vi "Topo & GridSpectr_DriftCorrection_zSpec_v18.vi"(6 "Internal use":string, 7 "Grid param":T1 {"height (m)" format="%#_6p"; "width (m)" format="%#_6p"; "center Y (m)" format="%#_6p"; "center X (m)" format="%#_6p"}, 8 "Error in (no error)":errorcluster, 9 "Points Y/Index Y":i32, 10 "Points X/Index X":i32, 11 "Method":enum16{"init", "run", "end"}(ring)=enum."end") -> (0 "Error out":errorcluster)   [LabVIEW 2014]
doc: "Example of a measurement VI to be used in the \"Experiments on a Grid\" tool as external VI.\n\nThis example measure the topography and spectroscopy data. The spectroscopy measurements are taken on a subgrid. The data are saved to a sxm and a binary file.\n\n- Nanonis Programming Interface -"
uses:
  <userlib>/Nanonis Prog Interface V5/Scan/Grid/GridPatternGet.vi
  <userlib>/Nanonis Prog Interface V5/Scan/Grid/LinePatternGet.vi
  <userlib>/Nanonis Prog Interface V5/Nanonis Prog Interface.lvlib
panel:
  in  "MultiGrid":bool
  in  "PLL ON/OFF":bool
  in  "Spectroscopy":u16(ring) items=["Bias", "zSpec"]
  in  "autoStop":bool
  in  "trigger 2 >Hz":sgl format="%#_6p"
  in  "trigger1 < Hz":sgl format="%#_6p"
  out "zFile":refnum<file>
  out "last z adjustment":sgl format="%#_6p"
  in  "during Spec Bias (V)":sgl format="%#_5p"
  in  "type":u16(ring)=1 items=["Line", "Grid"]
  in  "readjust setpoint every":i32=4
  in  "Correct Drift":bool=TRUE
  in  "Email when finished":string="cornelius.krull@monash.edu"
  in  "STS z offset":dbl format="%#_6p"
  out "ETA":timestamp
  out "remaining":dbl format="%<%H:%M:%S>t"
  out "Progress":u8(slide) scale=0.0..100.0 scale format="%#.1g"
  out "total Points":i32
  in  "preSTS delay [ms]":u32=500
  in  "ref Bias":dbl=0.02 format="%#_6p"
  in  "Imaging Bias":dbl=0.02 format="%#_6p"
  in  "max applied Drift Correction":i32=20 min=1 max=100 step=1 format="%.0p"
  in  "Correlate":u16(ring) items=["first Frame", "successive Frames"]
  out "Topo Images taken":i32=14
  in  "Increment":i32=40
  in  "Threshold":i32=2 min=1 step=1
  in  "tip Speed (m/s)":sgl=2e-09 format="%.2p"
  out "X drift":i32
  out "Y drift":i32
  out "Last Drift detected":i32=40
  in  "MaxImagesBack":i32=40
  in  "Channel index (0-23)":u8(ring) items=["Current"=0, "Z (m)"=14]
  in  "File name":string="symmetric_node"
  in  "ref Current":dbl=5e-12 format="%#_6p"
  in  "Imaging Current":dbl=5e-12 format="%#_6p"
  in  "zdrift \nDuration (s)":dbl
  in  "Correct z drift":bool
  out "Status":string="finishing"
  in  "Drift correction Pixels":i32=256 caption="Topo Pixels"
  out "Y Offset":dbl format="%#_6p"
  out "X Offset":dbl format="%#_6p"
  out "Points taken":dbl=14.0
  in  "Drift Correction every":i32=40
  # "z Spectroscopy"
  # "GRID points"
  # "Increase this if no Drift was detected for \na certain number of images"
  # "%"
  # "time (HH:MM:SS)"
  # "images back"
  # "% of image size"
  # "RUN smart tilt before starting the GRID\nImg Angle = 0\nmove tip to reference point for tip height"
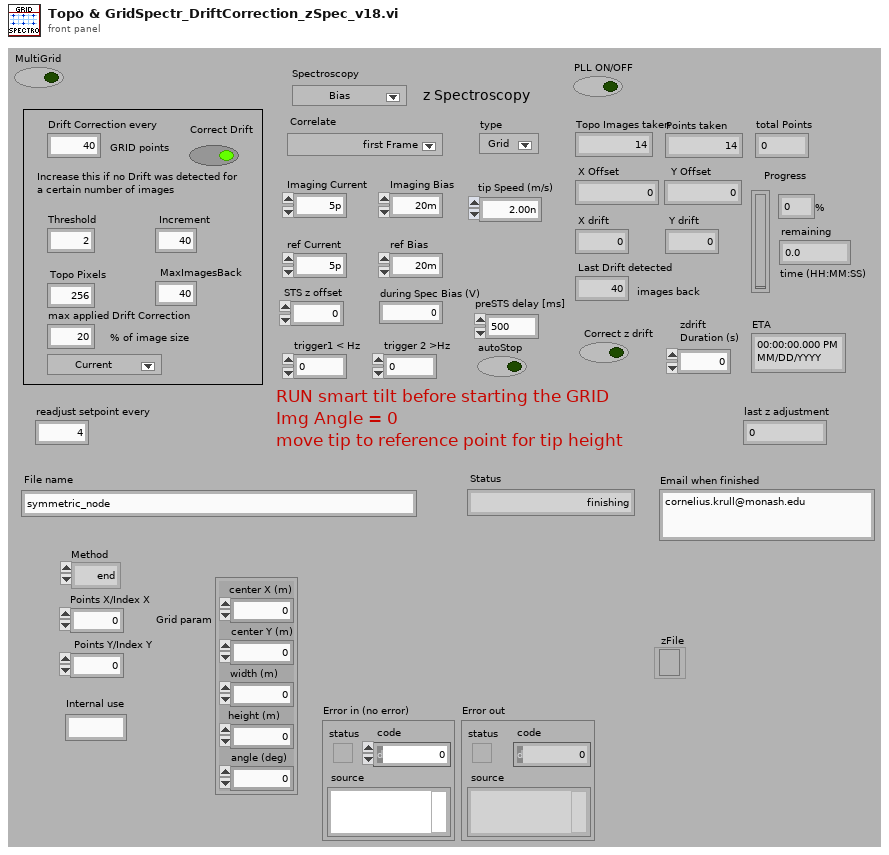
[diagram p1: front panel]
types:
  T1 = cluster{"center X (m)":sgl, "center Y (m)":sgl, "width (m)":sgl, "height (m)":sgl, "angle (deg)":sgl}
  T2 = enum16{"open", "replace", "create", "open or create", "replace or create", "replace or create with confirmation"}
  T3 = cluster{"Drift correction Pixels":i32, "Imaging Current":dbl, "STS Current":dbl, "MaxImagesBack":i32, "tip Speed (m/s)":sgl, "Threshold":i32, "Increment":i32, "Correlate":u16, "max applied Drift Correction":i32, "Imaging Bias":dbl, "Move Current":dbl, "Move Bias":dbl, "STS Bias":dbl, "preSTS delay [ms]":u32, "STS z offset":dbl, "Correct Drift":bool, "Lockin ON/OFF":bool}
  T4 = cluster{"x(m)":sgl, "y(m)":sgl, "Text":string, "Color":u32}
  T5 = cluster{"Z averaging time (s)":sgl, "Z offset (m)":sgl, "Initial settling time (s)":sgl}
  T6 = cluster{"center X":sgl, "center Y":sgl, "angle":sgl, "width":sgl, "height":sgl, "# pixels":i32, "# lines":i32}
  T7 = cluster{"Name":string, "Calibration":sgl, "Offset":sgl, "Channel index":i32}[]
  T8 = cluster{"up/down":bool, "time/line":sgl, "start time":timestamp, "end time":timestamp}
  T9 = cluster{"X (m)":sgl, "Y (m)":sgl, "Text":string, "Color":u32, "Visible":bool}[]
  T10 = cluster{"Max. slew rate (V/s)":sgl, "Settling time (s)":sgl, "Integration time (s)":sgl}
  T11 = cluster{"End settling time (s)":sgl, "Z control time (s)":sgl}
  T12 = cluster{"Z averaging time (s)":sgl, "Initial settling time (s)":sgl}
  T13 = cluster{"Max. slew rate (m/s)":sgl, "Settling time (s)":sgl, "Integration time (s)":sgl}
  T14 = cluster{"Points X/Index X":i32, "Points Y/Index Y":i32}
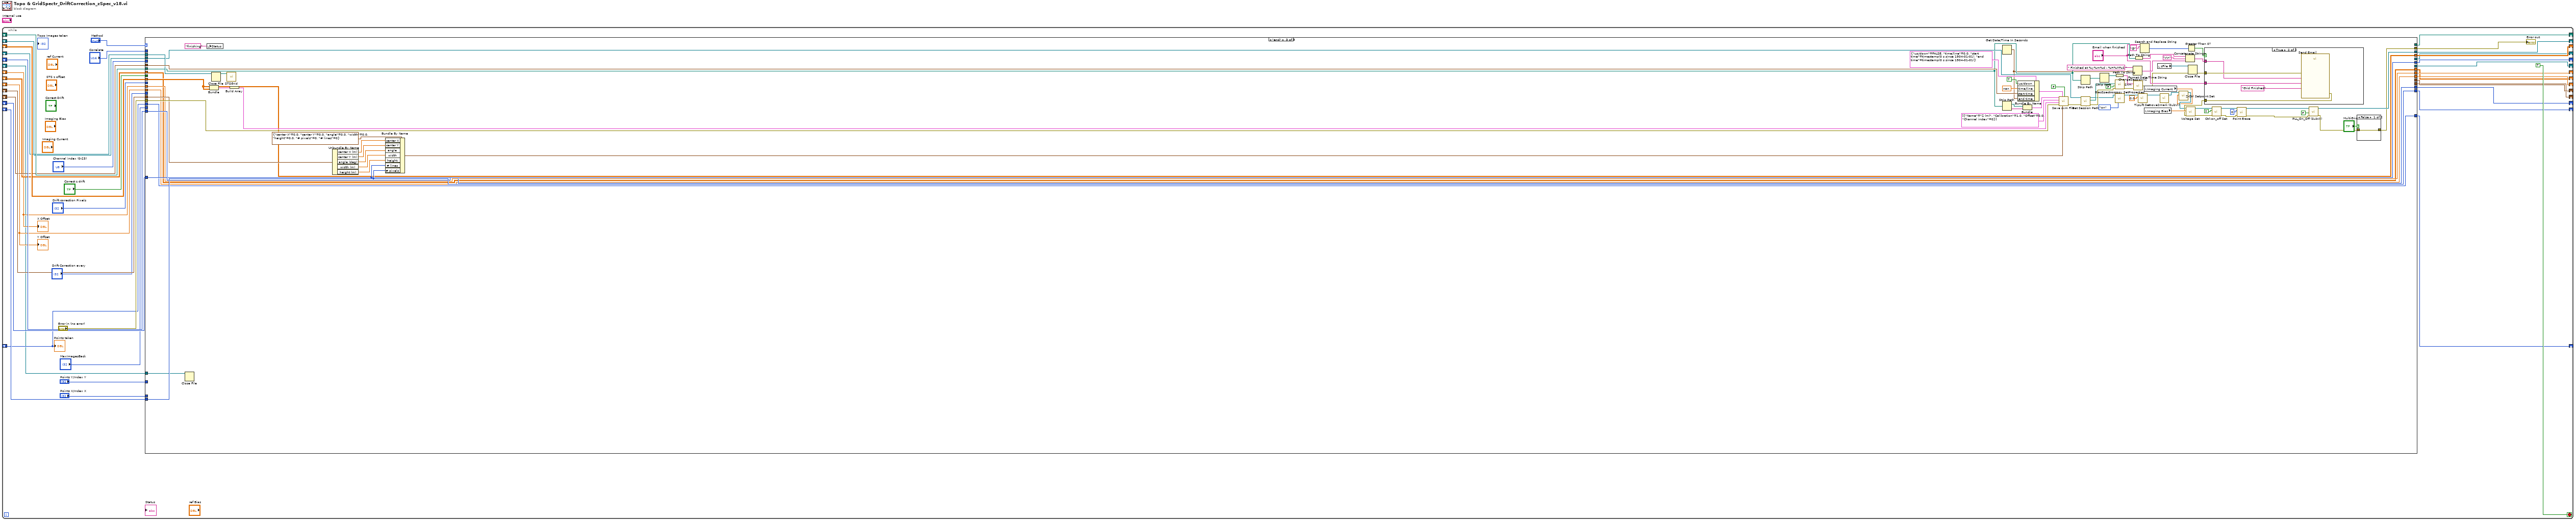
[diagram p0: block diagram]
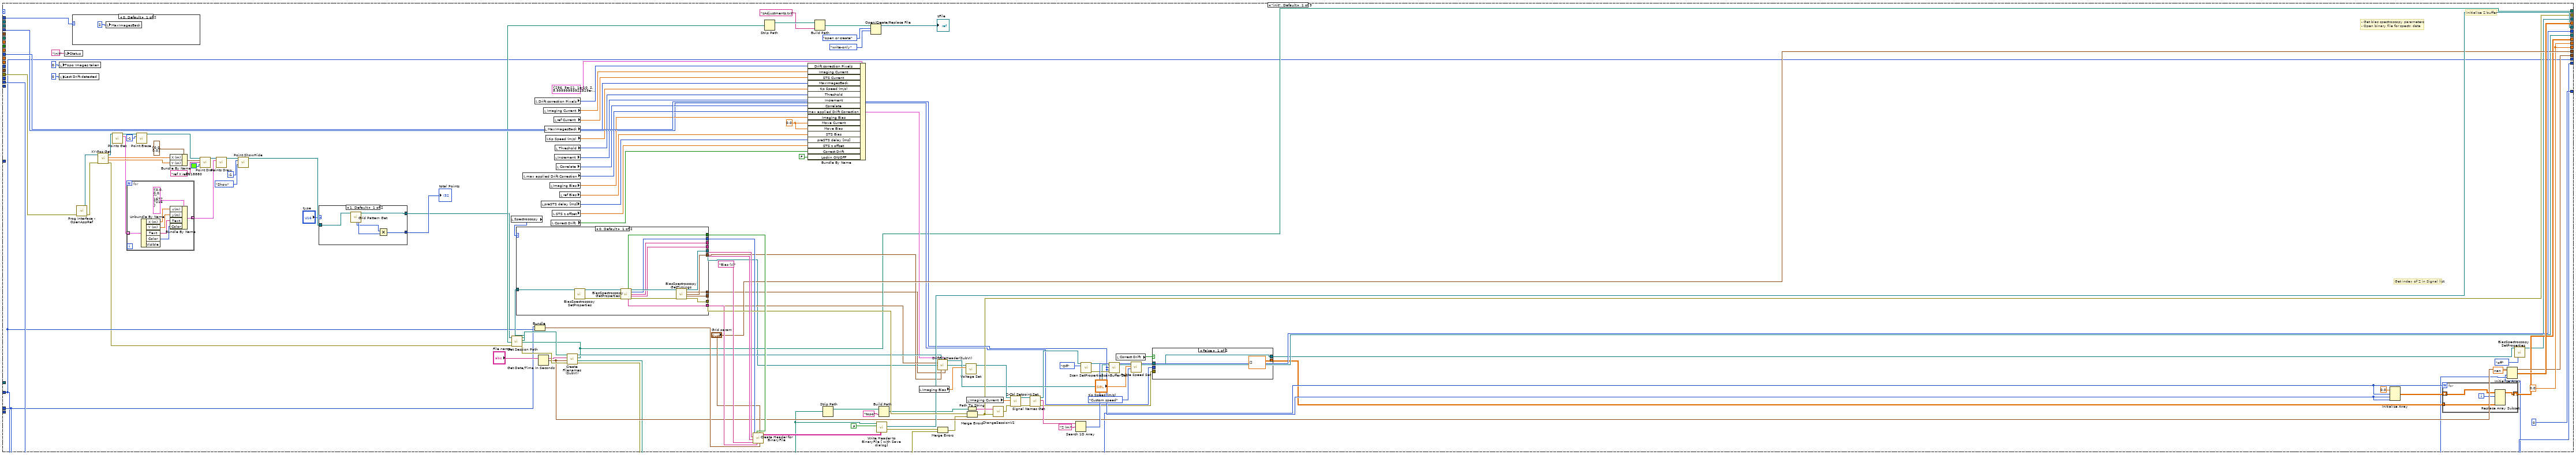
[diagram p2: hidden frame]
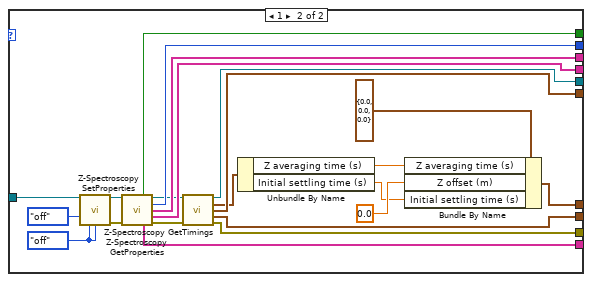
[diagram p3: hidden frame]
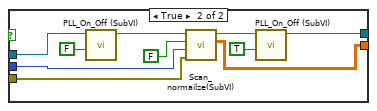
[diagram p4: hidden frame]
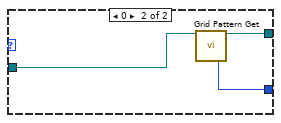
[diagram p5: hidden frame]
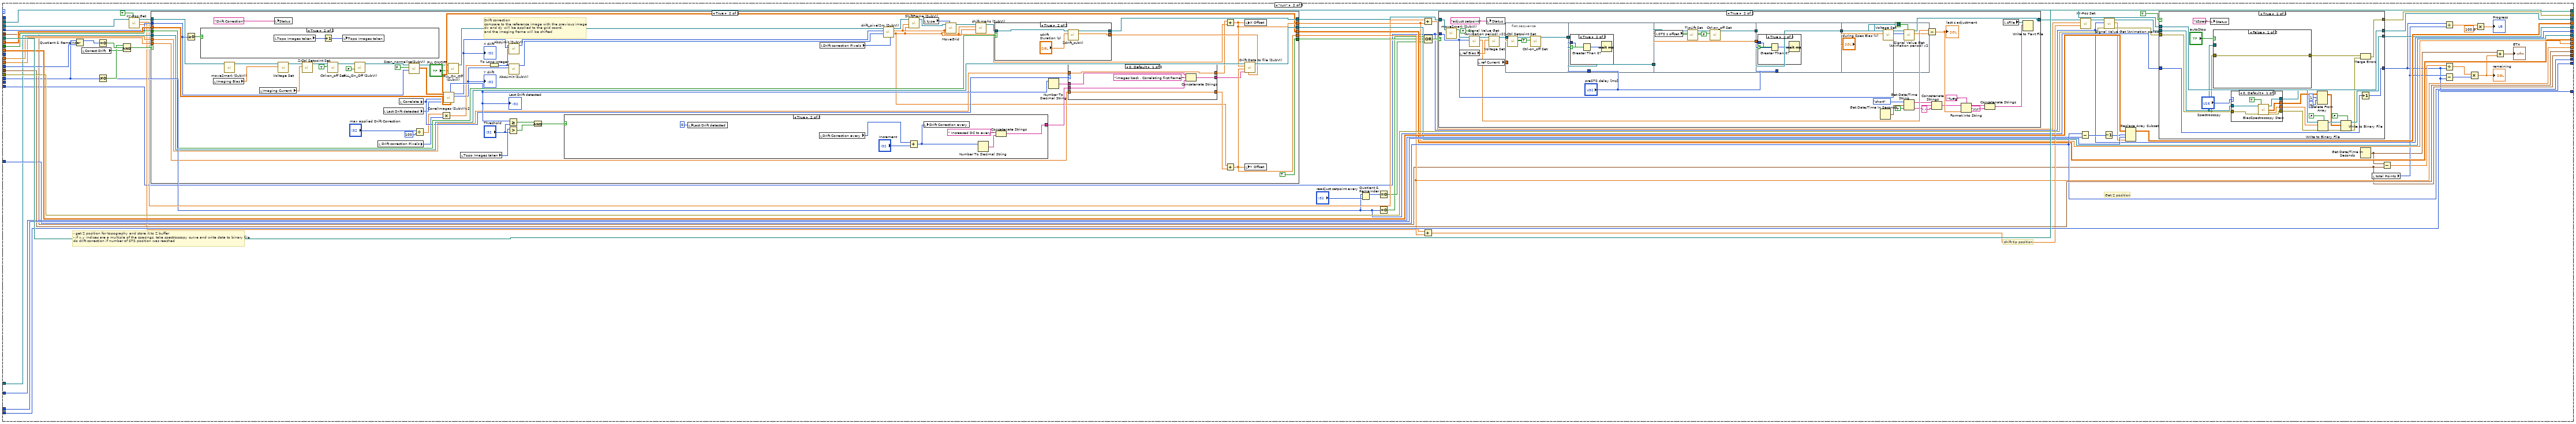
[diagram p7: hidden frame]
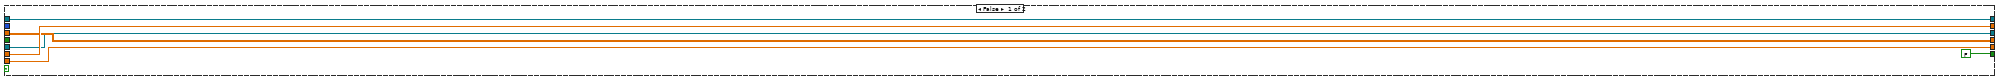
[diagram p11: hidden frame]
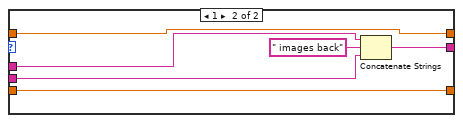
[diagram p12: hidden frame]
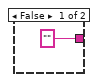
[diagram p14: hidden frame]
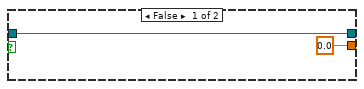
[diagram p15: hidden frame]
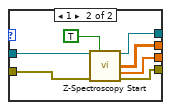
[diagram p17: hidden frame]
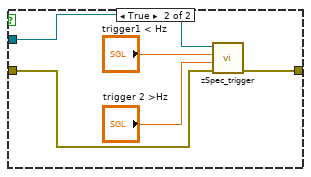
[diagram p18: hidden frame]
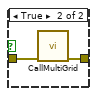
[diagram p19: hidden frame]
diagram:
  n1 = while {
    shift-right: [w21] -> _
    shift-left: _ -> [w38]
    shift-right: [w33] -> _
    shift-left: _ -> [w32]
    shift-right: [w30] -> _
    shift-left: _ -> [w31]
    shift-right: [w29] -> _
    shift-left: _ -> [w28]
    shift-right: [w27] -> _
    shift-left: _ -> [w26]
    shift-right: [w25] -> _
    shift-left: _ -> [w24]
    shift-right: [w23] -> _
    shift-left: _ -> [w22]
    shift-right: [w20] -> _
    shift-left: _ -> [w19]
    shift-right: [w18] -> _
    shift-left: _ -> [w17]
    shift-right: [w16] -> _
    shift-left: _ -> [w9]
    shift-right: [w15] -> _
    shift-left: _ -> [w8]
    shift-right: [w14] -> _
    shift-left: _ -> [w11]
    shift-right: [w13] -> _
    shift-left: _ -> [w10]
    shift-right: [w6] -> _
    shift-left: _ -> [w5]
    stop <- TRUE stop-if-true
    n2 = case shown="\"end\"" "Method" {
      tunnel: [w60 w296 _] -> w21
      tunnel: w38 -> [_ w296 w530]
      tunnel: "Error in (no error)" -> [w136 w289 w560]
      tunnel: [w116 w295 w498] -> w36
      tunnel: "Points X/Index X" -> [w53 w290 _]
      tunnel: "Points Y/Index Y" -> [w52 w283 _]
      tunnel: [w162 w293 w549] -> w33
      tunnel: w32 -> [_ w294 w549]
      tunnel: w31 -> [_ w292 w542]
      tunnel: [w154 w291 _] -> w30
      tunnel: [w152 w233 w572] -> w29
      tunnel: w28 -> [_ w233 w572]
      tunnel: [w105 w276 w507] -> w27
      tunnel: w26 -> [_ w260 w535]
      tunnel: ["Grid param" w286 _] -> w25
      tunnel: w24 -> [_ w286 w559]
      tunnel: [w134 w251 _] -> w23
      tunnel: w22 -> [_ w251 w567]
      tunnel: [w52 w284 w550] -> w20
      tunnel: w19 -> [_ w284 w550]
      tunnel: [w53 w285 w551] -> w18
      tunnel: w17 -> [_ w285 w551]
      tunnel: [w145 w266 w548] -> w16
      tunnel: [w145 w271 w546] -> w15
      tunnel: [w130 w265 w543] -> w14
      tunnel: [0 w249 w547] -> w13
      tunnel: w10 -> [_ w235 w547]
      tunnel: "Drift Correction every" -> [_ w279 _]
      tunnel: w11 -> [_ w270 w543]
      tunnel: w9 -> [_ w277 w548]
      tunnel: w8 -> [_ w263 w546]
      tunnel: "Drift correction Pixels" -> [w129 _ _]
      tunnel: [w102 w268 _] -> w6
      tunnel: w5 -> [_ w269 w544]
      tunnel: "Correct z drift" -> [_ w267 _]
      tunnel: "Channel index (0-23)" -> [w84 w264 _]
      tunnel: "MaxImagesBack" -> [w128 _ _]
      tunnel: "Correlate" -> [w112 _ _]
      frame "init", Default {
        w62 = 0.0 ("Move Current")
        w145 = 0.0
        # "- Get bias spectroscopy parameters\n- Open binary file for spectr. data"
        # "initialize Z buffer"
        # "Get index of Z in Signal list"
        n3 = local write "Topo Images taken"(0 ("Images taken")) -> ()
        n4 = local write "Last Drift detected"(0 ("Last Drift detected")) -> ()
        n5 = local write "Status"("init" ("Status")) -> ()
        n6 = case shown="0, Default" w112 {
          frame 0, Default {
            n7 = local write "MaxImagesBack"(2 ("StepsBack")) -> ()
          }
          frame 1 {
          }
        }
        n8 = call <userlib>:"Prog Interface - OpenAppRef.vi"("Error in (no error)"=w136) -> ("Error out"=w80:errorcluster, "Application reference"=w81:refnum<vi>)  [unwired: 5 in]
        n9 = call <userlib>:"XY-Pos Get.vi"("error in (no error)"=w80, "Application ref in"=w81) -> ("error out"=w49:errorcluster, "Y (m)"=w74:sgl, "X (m)"=w75:sgl, "Application ref out"=w45:refnum<vi>)  [unwired: 5 in]
        n10 = call <userlib>:"Points Get.vi"("Application ref in"=w45) -> ("Application ref out"=w44:refnum<vi>, "Points"=w46:T9)  [unwired: 12 in, 1 out]
        n11 = for {
          tunnel: w46 -> [w169] mode=indexing
          tunnel: [w163] -> w41 mode=indexing
          n12 = Unbundle By Name(w169) -> ("X (m)"=w167:sgl, "Y (m)"=w166:sgl, "Text"=w165:string, "Color"=w164:u32)  [unwired: 1 out]
          n13 = Bundle By Name(cluster=T4 {"x(m)"=0.0, "y(m)"=0.0, "Text"="", "Color"=16777216} ("Point"), "x(m)"=w167, "y(m)"=w166, "Text"=w165, "Color"=w164) -> (w163:T4)
        }
        n14 = call <userlib>:"Point Erase.vi"("Application ref in"=w44, "Point index (-1=All points)"=-1) -> ("Application ref out"=w67:refnum<vi>)  [unwired: 12 in, 1 out]
        n15 = Bundle By Name(cluster=cluster{"X (m)":sgl, "Y (m)":sgl} {"X (m)"=0.0, "Y (m)"=0.0} ("Point Coordinates"), "X (m)"=w75, "Y (m)"=w74) -> (w76:cluster{"X (m)":sgl, "Y (m)":sgl})
        n16 = call <userlib>:"Point Draw.vi"("Application ref in"=w67, "Point Coordinates"=w76, "Text"="ref X ref", "Color"=u32 6618880) -> ("Application ref out"=w43:refnum<vi>)  [unwired: 10 in, 1 out]
        n17 = call <userlib>:"Points Draw.vi"("Application ref in"=w43, "Points Configuration"=w41) -> ("Application ref out"=w42:refnum<vi>)  [unwired: 12 in, 1 out]
        n18 = call <userlib>:"Point ShowHide.vi"("Application ref in"=w42, "Point index (-1=All points)"=-1, "Show/Hide"=enum16{"Show", "Hide"}."Show") -> ("Application ref out"=w70:refnum<vi>)  [unwired: 11 in, 1 out]
        n19 = case shown="1, Default" "type" {
          tunnel: [w223 w226] -> w48
          tunnel: [w220 w224] -> w106
          tunnel: w70 -> [w219 w225]
          frame 1, Default {
            n20 = call-poly <userlib>:"Grid Pattern Get.vi"("Application ref in"=w219) -> ("Points Y"=w221:i32, "Points X"=w222:i32, "Application ref out"=w223:refnum<vi>)  [unwired: 10 in, 6 out]
            n21 = Multiply(x=w221, y=w222) -> (x*y=w220:i32)
          }
          frame 0 {
            n22 = call-poly <userlib>:"Grid Pattern Get.vi"("Application ref in"=w225) -> ("Points"=w224:i32, "Application ref out"=w226:refnum<vi>)  [unwired: 12 in, 5 out]
          }
        }
        "total Points" <- w106
        n23 = local read "Spectroscopy"() -> (w50:u16)
        n24 = call <userlib>:"Get Session Path.vi"("error in (no error)"=w49, "Application ref in"=w48) -> ("error out"=w135:errorcluster, "Session path"=w122:path, "Application ref out"=w114:refnum<vi>)  [unwired: 7 in]
        n25 = case shown="0, Default" w50 {
          tunnel: [w171 w206] -> w158
          tunnel: [w174 w205] -> w156
          tunnel: [w178 w192] -> w155
          tunnel: [w173 w204] -> w151
          tunnel: [w172 w203] -> w149
          tunnel: [w175 w202] -> w148
          tunnel: w114 -> [w180 w195]
          tunnel: [w177 w200] -> w73
          tunnel: [w176 w199] -> w72
          tunnel: [w170 w185] -> w47
          tunnel: [w179 w198] -> w51
          frame 0, Default {
            n26 = call <userlib>:"BiasSpectroscopy SetProperties.vi"("Application ref in"=w180) -> ("Application ref out"=w184:refnum<vi>, "Error out"=w183:errorcluster)  [unwired: 13 in]
            n27 = call <userlib>:"BiasSpectroscopy GetProperties.vi"("Application ref in"=w184, "Error in (no error)"=w183) -> ("Backward sweep"=w171:bool, "Application ref out"=w182:refnum<vi>, "Number of points"=w172:i32, "Channels"=w175:string[], "Parameters"=w174:string[], "Fixed parameters"=w173:string[], "Error out"=w181:errorcluster)  [unwired: 5 in, 2 out]
            n28 = call <userlib>:"BiasSpectroscopy GetTimings.vi"("Application ref in"=w182, "Error in (no error)"=w181) -> ("Application ref out"=w179:refnum<vi>, "Initialization"=w170:T5, "Sweep Timing"=w176:T10, "End of Sweep"=w177:T11, "Error out"=w178:errorcluster)  [unwired: 9 in]
          }
          frame 1 {
            w197 = enum16{"no change", "on", "off"}."off" ("Save dialog")
            n29 = call <userlib>:"Z-Spectroscopy SetProperties.vi"("Application ref in"=w195, "Autosave"=enum16{"no change", "on", "off"}."off" ("Autosave (no change)"), "Save dialog"=w197, "Save all sweeps (no change)"=w197) -> ("Application ref out"=w194:refnum<vi>, "error out"=w193:errorcluster)  [unwired: 10 in]
            n30 = call <userlib>:"Z-Spectroscopy GetProperties.vi"("Application ref in"=w194, "error in (no error)"=w193) -> ("Backward sweep"=w206:bool, "Application ref out"=w201:refnum<vi>, "Number of points"=w203:i32, "Channels"=w202:string[], "Parameters"=w205:string[], "Fixed parameters"=w204:string[], "error out"=w191:errorcluster)  [unwired: 6 in, 1 out]
            n31 = call <userlib>:"Z-Spectroscopy GetTimings.vi"("Application ref in"=w201, "Error in (no error)"=w191) -> ("Application ref out"=w198:refnum<vi>, "Initialization"=w186:T12, "Sweep Timing"=w199:T13, "End of Sweep"=w200:T11, "Error out"=w192:errorcluster)  [unwired: 9 in]
            n32 = Unbundle By Name(w186) -> ("Z averaging time (s)"=w188:sgl, "Initial settling time (s)"=w189:sgl)
            n33 = Bundle By Name(cluster=T5 {"Z averaging time (s)"=0.0, "Z offset (m)"=0.0, "Initial settling time (s)"=0.0} ("Initialization"), "Z averaging time (s)"=w188, "Z offset (m)"=sgl 0.0, "Initial settling time (s)"=w189) -> (w185:T5)
          }
        }
        n34 = local read "max applied Drift Correction"() -> (w90:i32)
        n35 = local read "Drift correction Pixels"() -> (w98:i32)
        n36 = Bundle("Points X/Index X"=w53, "Points Y/Index Y"=w52) -> (w157:T14)  [unwired: 1 in]
        n37 = Get Date/Time In Seconds() -> (seconds since 1Jan1904=w134:timestamp)
        n38 = local read "preSTS delay [ms]"() -> (w87:u32)
        n39 = local read "Imaging Current"() -> (w97:dbl)
        n40 = local read "MaxImagesBack"() -> (w94:i32)
        n41 = local read "tip Speed (m/s)"() -> (w95:sgl)
        n42 = local read "Imaging Bias"() -> (w89:dbl)
        n43 = local read "Correct Drift"() -> (w85:bool)
        n44 = local read "STS z offset"() -> (w86:dbl)
        n45 = local read "ref Current"() -> (w96:dbl)
        n46 = local read "Increment"() -> (w92:i32)
        n47 = local read "Threshold"() -> (w93:i32)
        n48 = local read "Correlate"() -> (w91:u16)
        n49 = local read "ref Bias"() -> (w88:dbl)
        n50 = call "Create Filenames (SubVI).vi"("error in (no error)"=w135, "seconds since 1Jan1904"=w134, "File name"="File name", "Session path"=w122) -> ("error out"=w125:errorcluster, "binFilePath"=w118:path, "topoFilePath"=w60:path, "Drift File out"=w103:refnum<file>)  [unwired: 4 in]
        n51 = call <userlib>:"Create Header for BinaryFile.vi"("Grid points"=w157, "Grid param"="Grid param", "Fixed parameters"=w151, "Backward sweep"=w158, "Sweep signal"="Bias (V)" ("Sweep Signal"), "Parameters"=w156, "Channels"=w148, "Points per sweep"=w149) -> ("Header (fixed attributes)"=w160:string[][])  [unwired: 3 in]
        n52 = Strip Path(path=w60) -> (stripped path=w59:path)  [unwired: 1 out]
        n53 = Bundle By Name(cluster=T3 {"Drift correction Pixels"=256, "Imaging Current"=5e-11, "STS Current"=1e-10, "MaxImagesBack"=2, "tip Speed (m/s)"=1e-08, "Threshold"=2, "Increment"=64, "Correlate"=0, "max applied Drift Correction"=20, "Imaging Bias"=-0.02, "Move Current"=1.5e-11, "Move Bias"=-0.02, "STS Bias"=0.1, "preSTS delay [ms]"=1000, "STS z offset"=-1.7e-10, "Correct Drift"=TRUE, "Lockin ON/OFF"=TRUE} ("Drift Correction"), "Drift correction Pixels"=w98, "Imaging Current"=w97, "STS Current"=w96, "MaxImagesBack"=w94, "tip Speed (m/s)"=w95, "Threshold"=w93, "Increment"=w92, "Correlate"=w91, "max applied Drift Correction"=w90, "Imaging Bias"=w89, "Move Current"=w62, "Move Bias"=w62, "STS Bias"=w88, "preSTS delay [ms]"=w87, "STS z offset"=w86, "Correct Drift"=w85, "Lockin ON/OFF"=FALSE) -> (w100:T3)
        n54 = Build Path(base path=w59, name or relative path="zAdjustments.txt") -> (appended path=w57:path)
        n55 = Strip Path(path=w118) -> (stripped path=w121:path)  [unwired: 1 out]
        n56 = Open/Create/Replace File(file path (use dialog)=w57, operation (0:open)=T2."open or create", access (0:read/write)=enum16{"read/write", "read-only", "write-only"}."write-only") -> (refnum out=→"zFile":refnum<file>)  [unwired: 3 in, 2 out]
        n57 = call <userlib>:"Write Header to BinaryFile [ with Save dialog].vi"("Fixed Attributes"=w160, "Show Dialog? (T)"=FALSE, "Filename"=w118) -> ("Error out"=w126:errorcluster, "File ref"=w154:refnum<file>)  [unwired: 5 in, 2 out]
        n58 = Build Path(base path=w121, name or relative path="topo") -> (appended path=w119:path)
        n59 = local read "Imaging Bias"() -> (w108:dbl)
        n60 = call "DriftFileHeader(SubVI).vi"("Byte Stream File in"=w103, "Drift Correction"=w100, "End of Sweep"=w73, "Application ref in"=w51, "Sweep Timing"=w72, "Initialization"=w47) -> ("Byte Stream File out"=w102:refnum<file>, "Application ref out"=w101:refnum<vi>)  [unwired: 8 in]
        n61 = Merge Errors(w126, w125) -> (w127:errorcluster)
        n62 = call <userlib>:"Voltage Set.vi"("Bias (V)"=w108, "Application ref in"=w101) -> ("Application ref out"=w109:refnum<vi>)  [unwired: 8 in, 1 out]
        n63 = local read "Imaging Current"() -> (w107:dbl)
        n64 = Path To String(path=w119) -> (string=w117:string)
        n65 = Merge Errors(w155, w127) -> (w116:errorcluster)
        n66 = call "ChangeSessionV2.vi"("error in (no error)"=w116, "Session"=w117) -> ("error out"=w115:errorcluster)
        n67 = call <userlib>:"Z-Ctrl Setpoint Set.vi"("error in (no error)"=w115, "Z Controller setpoint"=w107, "Application ref in"=w109) -> ("error out"=w137:errorcluster, "Application ref out"=w138:refnum<vi>)  [unwired: 7 in]
        n68 = call <userlib>:"Signal Names Get.vi"("error in (no error)"=w137, "Application ref in"=w138) -> ("error out"=w83:errorcluster, "Signals Names"=w150:string[], "Application ref out"=w141:refnum<vi>)  [unwired: 5 in]
        n69 = Search 1D Array(1D array=w150, element="Z (m)") -> (index of element=w152:i32)  [unwired: 1 in]
        n70 = call <userlib>:"Scan SetProperties.vi"("Application ref in"=w141, "Continuous scan"=enum16{"No change", "On", "Off"}."Off") -> ("Application ref out"=w143:refnum<vi>, "Error out"=w142:errorcluster)  [unwired: 12 in]
        n71 = call <userlib>:"ScanBuffer Set.vi"("Application ref in"=w143, "Pixels"=w129, "Lines"=w129, "error in (no error)"=w142) -> ("Application ref out"=w110:refnum<vi>)  [unwired: 10 in, 1 out]
        n72 = local read "Correct Drift"() -> (w63:bool)
        n73 = call <userlib>:"FolMe Speed Set.vi"("Speed Setting (Custom)"=enum32{"Scan speed", "Custom speed"}."Custom speed", "Speed (m/s)"="tip Speed (m/s)", "Application ref in"=w110) -> ("Application ref out"=w65:refnum<vi>)  [unwired: 5 in, 1 out]
        n74 = case shown="False" w63 {
          tunnel: w84 -> [_ w218]
          tunnel: w83 -> [_ w217]
          tunnel: [dbl[][] [] ("Array") w216] -> w82
          tunnel: w65 -> [w208 w214]
          tunnel: [w208 w209] -> w61
          frame False {
          }
          frame True {
            n75 = call "PLL_On_Off (SubVI).vi"("Output ON/OFF (F=OFF)"=FALSE, "Application in"=w214) -> ("Application out"=w213:refnum<vi>)  [unwired: 8 in, 1 out]
            n76 = call "Scan_normailze(SubVI).vi"("error in (no error)"=w217, "Channel index (0-23)"=w218, "Normalization"=FALSE ("Boolean"), "Application in"=w213) -> ("Array"=w216:dbl[][], "Application out"=w210:refnum<vi>)  [unwired: 5 in, 1 out]
            n77 = call "PLL_On_Off (SubVI).vi"("Output ON/OFF (F=OFF)"=TRUE, "Application in"=w210) -> ("Application out"=w209:refnum<vi>)  [unwired: 8 in, 1 out]
          }
        }
        n78 = Initialize Array(0.0 ("element"), w128, w129, w129) -> (w131:dbl[][][])
        n79 = for {
          N: w128 -> [_]
          tunnel: w82 -> [w230]
          shift-right: [w229] -> w130
          shift-left: w131 -> [w231]
          i -> [w228]
          n80 = Replace Array Subset(array=w231, new element=w230, index (dim 0)=w228) -> (w229:dbl[][][])  [unwired: 2 in]
        }
        n81 = Initialize Array(sgl nan ("element"), w52, w53) -> (w162:sgl[][])
        n82 = call <userlib>:"BiasSpectroscopy SetProperties.vi"("Application ref in"=w61, "Z-Controller hold (no change)"=enum16{"no change", "on", "off"}."off") -> ("Application ref out"=w105:refnum<vi>)  [unwired: 12 in, 1 out]
      }
      frame "run" {
        # "shift tip position"
        # "Get Z position"
        # "- get Z position for topography and store it to Z buffer\n- if x,y indices are a multiple of the spacings, take spectroscopy curve and write data to binary file\ndo drift correction if number of STS position was reached"
        n83 = Quotient & Remainder(x=w235, y=w279) -> (x-y*floor(x/y)=w280:i32)  [unwired: 1 out]
        n84 = local read "Correct Drift"() -> (w243:bool)
        n85 = Equal To 0?(x=w280) -> (x = 0?=w278:bool)
        n86 = Not Equal To 0?(x=w235) -> (x != 0?=w261:bool)
        n87 = Compound Arithmetic op=AND(w261, w278, w243) -> (w262:bool)
        n88 = call <userlib>:"XY-Pos Get.vi"("Wait for newest data (F=False)"=TRUE, "Application ref in"=w260) -> ("Y (m)"=w256:sgl, "X (m)"=w257:sgl, "Application ref out"=w259:refnum<vi>)  [unwired: 5 in, 1 out]
        n89 = case shown="True" w262 {
          tunnel: w259 -> [w357 w369]
          tunnel: [w357 w414] -> w240
          tunnel: w270 -> [w354 w410]
          tunnel: [w356 w412] -> w266
          tunnel: [w355 w411] -> w271
          tunnel: w277 -> [w356 w393]
          tunnel: w263 -> [w355 w391]
          tunnel: [w354 w406] -> w265
          tunnel: w269 -> [w353 w417]
          tunnel: [w353 w416] -> w268
          tunnel: w267 -> [_ w413]
          tunnel: w264 -> [_ w397]
          tunnel: [FALSE TRUE] -> w237
          frame False {
          }
          frame True {
            # "Drift correction \ncompare to the reference image with the previous image \ndx and dy will be applied to the grid coord, \nand the imaging frame will be shifted"
            n90 = Greater Or Equal To 0?(x=w397) -> (x >= 0?=w396:bool)
            n91 = case shown="True" w396 {
              frame False {
              }
              frame True {
                n92 = local read "Topo Images taken"() -> (w432:i32)
                n93 = Increment(x=w432) -> (x+1=w431:i32)
                n94 = local write "Topo Images taken"(w431) -> ()
              }
            }
            n95 = local read "Imaging Bias"() -> (w376:dbl)
            n96 = call "move2mark (SubVI).vi"("Application in"=w369) -> ("Application out"=w368:refnum<vi>)  [unwired: 10 in]
            n97 = local read "Imaging Current"() -> (w375:dbl)
            n98 = local write "Status"("Drift Correction" ("Status")) -> ()
            n99 = call <userlib>:"Voltage Set.vi"("Bias (V)"=w376, "Application ref in"=w368) -> ("Application ref out"=w377:refnum<vi>)  [unwired: 8 in, 1 out]
            n100 = call <userlib>:"Z-Ctrl Setpoint Set.vi"("Z Controller setpoint"=w375, "Application ref in"=w377) -> ("Application ref out"=w367:refnum<vi>)  [unwired: 8 in, 1 out]
            n101 = call <userlib>:"Ctrl-on_off Set.vi"("Z Controller ON/OFF"=TRUE, "Application ref in"=w367) -> ("Application ref out"=w365:refnum<vi>)  [unwired: 8 in, 1 out]
            n102 = call "PLL_On_Off (SubVI).vi"("Output ON/OFF (F=OFF)"=FALSE, "Application in"=w365) -> ("Application out"=w364:refnum<vi>)  [unwired: 8 in, 1 out]
            n103 = local read "Drift correction Pixels"() -> (w385:i32)
            n104 = local read "Last Drift detected"() -> (w388:i32)
            n105 = local read "Correlate"() -> (w394:u16)
            n106 = call "Scan_normailze(SubVI).vi"("Channel index (0-23)"=w397, "Normalization"=FALSE ("Boolean"), "Application in"=w364) -> ("Array"=w407:dbl[][], "Application out"=w362:refnum<vi>)  [unwired: 6 in, 1 out]
            n107 = Divide(x="max applied Drift Correction", y=100) -> (x/y=w384:dbl)
            n108 = Multiply(x=w384, y=w385) -> (x*y=w386:dbl)
            n109 = call "CorrelImages (SubVI)v2.vi"("last drift detected"=w388, "Correlate"=w394, "Ref Array"=w410, "New Image"=w407) -> ("Y drift"=w382:i32, "X drift"=w379:i32, "Ref Array out"=w406:dbl[][][], "Queue Steps"=w395:i32)  [unwired: 4 in]
            "X drift" <- w379
            "Y drift" <- w382
            "Last Drift detected" <- w395
            n110 = call "PLL_On_Off (SubVI).vi"("Output ON/OFF (F=OFF)"="PLL ON/OFF", "Application in"=w362) -> ("Application out"=w360:refnum<vi>)  [unwired: 8 in, 1 out]
            n111 = local read "Topo Images taken"() -> (w399:i32)
            n112 = To Long Integer(number=w386) -> (32bit integer=w378:i32)
            n113 = Greater Or Equal?(x=w395, y="Threshold") -> (x >= y?=w401:bool)
            n114 = Greater?(x=w399, y="Threshold") -> (0:w398:bool)
            n115 = call "AbsLimit (SubVI).vi"("in"=w379, "Abslimt"=w378) -> ("Numeric out"=w381:i32)  [unwired: 9 in]
            n116 = call "AbsLimit (SubVI).vi"("in"=w382, "Abslimt"=w378) -> ("Numeric out"=w380:i32)  [unwired: 9 in]
            n117 = And(x=w401, y=w398) -> (x .and. y?=w400:bool)
            n118 = case shown="True" w400 {
              tunnel: ["" w436] -> w402
              frame False {
              }
              frame True {
                n119 = local write "Last Drift detected"(0 ("Last Drift detected")) -> ()
                n120 = local read "Drift Correction every"() -> (w435:i32)
                n121 = Add(x=w435, y="Increment") -> (x+y=w439:i32)
                n122 = local write "Drift Correction every"(w439) -> ()
                n123 = Number To Decimal String(number=w439) -> (decimal integer string=w438:string)  [unwired: 1 in]
                n124 = Concatenate Strings(" Increased DC to every " ("string"), w438) -> (w436:string)
              }
            }
            n125 = local read "Drift correction Pixels"() -> (w404:i32)
            n126 = call "drift_pixel2m (SubVI).vi"("Application in"=w360, "X drift"=w381, "Y drift"=w380, "Drift correction Pixels"=w404) -> ("Application out"=w403:refnum<vi>, "x drift"=w373:sgl, "y drift"=w372:sgl)  [unwired: 2 in, 1 out]
            n127 = call "ShiftFrame (SubVI).vi"("Y shift"=w372, "X shift"=w373, "Application in"=w403) -> ("Application out"=w405:refnum<vi>)  [unwired: 8 in]
            n128 = local read "type"() -> (w359:u16)
            n129 = call "MoveGrid.vi"("type"=w359, "y"=w372, "x"=w373, "Application ref in"=w405) -> ("Application ref out"=w371:refnum<vi>)  [unwired: 6 in, 1 out]
            n130 = call "shift marks (SubVI).vi"("y"=w372, "x"=w373, "Application in"=w371) -> ("Application out"=w370:refnum<vi>)  [unwired: 7 in, 1 out]
            n131 = case shown="True" w413 {
              tunnel: [0.0 ("z drift") w446] -> w415
              tunnel: w370 -> [w441 w445]
              tunnel: [w441 w444] -> w414
              frame False {
              }
              frame True {
                n132 = call "Zdrift_subVi.vi"("Duration"="zdrift \nDuration (s)", "Application in"=w445) -> ("z drift"=w446:dbl, "Application out"=w444:refnum<vi>)  [unwired: 7 in, 1 out]
              }
            }
            n133 = Number To Decimal String(number=w395) -> (decimal integer string=w409:string)  [unwired: 1 in]
            n134 = case shown="0, Default" w394 {
              tunnel: w409 -> [w419 w430]
              tunnel: [w424 w429] -> w408
              tunnel: w402 -> [w422 w427]
              tunnel: w393 -> [w420 w426]
              tunnel: [w420 w426] -> w392
              tunnel: w391 -> [w421 w425]
              tunnel: [w421 w425] -> w390
              frame 0, Default {
                n135 = Concatenate Strings(w419, "images back , Correlating first frame " ("string"), w422) -> (w424:string)
              }
              frame 1 {
                n136 = Concatenate Strings(w430, " images back" ("string"), w427) -> (w429:string)
              }
            }
            n137 = Add(x=w392, y=w373) -> (x+y=w412:dbl)
            n138 = Add(x=w372, y=w390) -> (x+y=w411:dbl)
            n139 = local write "X Offset"(w412) -> ()
            n140 = call "Drift Data to file (SubVI).vi"("z drift"=w415, "Comment"=w408, "y Drift"=w411, "X drift"=w412, "Byte Stream File in"=w417) -> ("Byte Stream File out"=w416:refnum<file>)  [unwired: 6 in]
            n141 = local write "Y Offset"(w411) -> ()
          }
        }
        n142 = Quotient & Remainder(x=w235, y="readjust setpoint every") -> (x-y*floor(x/y)=w236:i32)  [unwired: 1 out]
        n143 = Equal To 0?(x=w236) -> (x = 0?=w239:bool)
        n144 = Equal To 0?(x=w235) -> (x = 0?=w234:bool)
        n145 = Add(x=w257, y=w266) -> (x+y=w273:dbl)
        n146 = Add(x=w256, y=w271) -> (x+y=w272:dbl)
        n147 = Compound Arithmetic op=OR(w234, w237, w239) -> (w238:bool)
        n148 = case shown="True" w238 {
          tunnel: [w297 w314] -> w241
          tunnel: w240 -> [w297 w330]
          tunnel: w233 -> [_ w316]
          frame False {
          }
          frame True {
            n149 = call "move2mark (SubVI).vi"("Application in"=w330) -> ("Application out"=w319:refnum<vi>)  [unwired: 10 in]
            n150 = local read "ref Bias"() -> (w329:dbl)
            n151 = call <userlib>:"Signal Value Get (Animation period) v2.vi"("Wait for newest data (F=False)"=TRUE, "Signal index (0-79)"=w316, "Application ref in"=w319) -> ("Signal value"=w312:sgl, "Application ref out"=w318:refnum<vi>)  [unwired: 5 in, 1 out]
            n152 = local read "ref Current"() -> (w326:dbl)
            n153 = local write "Status"("adjust setpoint" ("Status")) -> ()
            n154 = call <userlib>:"Voltage Set.vi"("Bias (V)"=w329, "Application ref in"=w318) -> ("Application ref out"=w327:refnum<vi>)  [unwired: 8 in, 1 out]
            n155 = flat-sequence {
              tunnel: w327 -> [w335]
              tunnel: [w332] -> w325
              tunnel: w326 -> [w334]
              tunnel: w325 -> [w338]
              tunnel: [w338] -> w324
              tunnel: "preSTS delay [ms]" -> [w336]
              tunnel: w324 -> [w343]
              tunnel: [w340] -> w328
              tunnel: [w341] -> w322
              tunnel: w328 -> [w347]
              tunnel: "preSTS delay [ms]" -> [w346]
              tunnel: w322 -> [_]
              tunnel: [w347] -> w320
              tunnel: [w349] -> w315
              tunnel: w320 -> [w350]
              frame #0 {
                n156 = call <userlib>:"Z-Ctrl Setpoint Set.vi"("Z Controller setpoint"=w334, "Application ref in"=w335) -> ("Application ref out"=w333:refnum<vi>)  [unwired: 8 in, 1 out]
                n157 = call <userlib>:"Ctrl-on_off Set.vi"("Z Controller ON/OFF"=TRUE, "Application ref in"=w333) -> ("Application ref out"=w332:refnum<vi>)  [unwired: 8 in, 1 out]
              }
              frame #1 {
                n158 = Greater Than 0?(x=w336) -> (x > 0?=w337:bool)
                n159 = case shown="True" w337 {
                  tunnel: w336 -> [_ w339]
                  frame False {
                  }
                  frame True {
                    n160 = Wait (ms)(milliseconds to wait=w339) -> ()  [unwired: 1 out]
                  }
                }
              }
              frame #2 {
                n161 = local read "STS z offset"() -> (w341:dbl)
                n162 = call <userlib>:"TipLift Set.vi"("TipLift (m)"=w341, "Application ref in"=w343) -> ("Application ref out"=w342:refnum<vi>)  [unwired: 8 in, 1 out]
                n163 = call <userlib>:"Ctrl-on_off Set.vi"("Z Controller ON/OFF"=FALSE, "Application ref in"=w342) -> ("Application ref out"=w340:refnum<vi>)  [unwired: 8 in, 1 out]
              }
              frame #3 {
                n164 = Greater Than 0?(x=w346) -> (x > 0?=w345:bool)
                n165 = case shown="True" w345 {
                  tunnel: w346 -> [_ w348]
                  frame False {
                  }
                  frame True {
                    n166 = Wait (ms)(milliseconds to wait=w348) -> ()  [unwired: 1 out]
                  }
                }
              }
              frame #4 {
                n167 = call <userlib>:"Voltage Set.vi"("Bias (V)"="during Spec Bias (V)", "Application ref in"=w350) -> ("Application ref out"=w349:refnum<vi>)  [unwired: 8 in, 1 out]
              }
            }
            n168 = Get Date/Time In Seconds() -> (seconds since 1Jan1904=w303:timestamp)
            n169 = call <userlib>:"Signal Value Get (Animation period) v2.vi"("Wait for newest data (F=False)"=TRUE, "Signal index (0-79)"=w316, "Application ref in"=w315) -> ("Signal value"=w311:sgl, "Application ref out"=w314:refnum<vi>)  [unwired: 5 in, 1 out]
            n170 = Get Date/Time String(date format (0)=enum16{"short", "long", "abbreviated"}."short", seconds (now)=w303, want seconds? (F)=TRUE) -> (date string=w307:string, time string=w306:string)
            n171 = Subtract(x=w312, y=w311) -> (x-y=w309:sgl)
            "last z adjustment" <- w309
            n172 = Concatenate Strings(w307, w306, "," ("string")) -> (w305:string)
            n173 = Format Into String(format string="%#g", initial string=w305, w309) -> (resulting string=w300:string)  [unwired: 1 in, 1 out]
            n174 = Concatenate Strings(w300, "\r\n") -> (w299:string)
            n175 = local read "zFile"() -> (w310:refnum<file>)
            n176 = Write to Text File(file (use dialog)=w310, text=w299) -> ()  [unwired: 2 in, 3 out]
          }
        }
        n177 = Subtract(x=w284, y=w283) -> (x-y=w282:i32)
        n178 = call <userlib>:"XY-Pos Set.vi"("Y (m)"=w272, "X (m)"=w273, "Application ref in"=w241) -> ("Application ref out"=w274:refnum<vi>)  [unwired: 5 in, 1 out]
        n179 = Decrement(x=w282) -> (x-1=w281:i32)
        n180 = call <userlib>:"Signal Value Get (Animation period).vi"("error in (no error)"=w289, "Signal index (0-47)"=w233, "Application ref in"=w274) -> ("error out"=w288:errorcluster, "Signal value"=w287:sgl, "Application ref out"=w275:refnum<vi>)  [unwired: 5 in]
        n181 = Replace Array Subset(array=w294, new element=w287, index (row)=w281, index (col)=w290) -> (w293:sgl[][])
        n182 = case shown="True" TRUE {
          tunnel: [w449 w453] -> w295
          tunnel: w292 -> [w450 w473]
          tunnel: [w450 w471] -> w291
          tunnel: w288 -> [w449 w456]
          tunnel: w275 -> [w448 w457]
          tunnel: [w448 w458] -> w276
          tunnel: [w447 w460] -> w249
          tunnel: w235 -> [w447 w461]
          frame False {
            # "Point indices aren't multiple of subgrid spacing\n=> no spectroscopy at this point"
          }
          frame True {
            n183 = local write "Status"("zSpec" ("Status")) -> ()
            n184 = case shown="False" "autoStop" {
              tunnel: w457 -> [_ w493]
              tunnel: w456 -> [w488 w490]
              tunnel: [w488 w489] -> w455
              frame False {
              }
              frame True {
                n185 = call "zSpec_trigger.vi"("Error in (no error)"=w490, "trigger 2"="trigger 2 >Hz", "trigger1"="trigger1 < Hz", "Application ref in"=w493) -> ("Error out"=w489:errorcluster)  [unwired: 5 in, 1 out]
              }
            }
            n186 = case shown="0, Default" "Spectroscopy" {
              tunnel: [w474 w487] -> w470
              tunnel: [w475 w486] -> w469
              tunnel: [w476 w484] -> w463
              tunnel: [w477 w483] -> w458
              tunnel: w457 -> [w479 w482]
              tunnel: w456 -> [w478 w481]
              frame 0, Default {
                n187 = call <userlib>:"BiasSpectroscopy Start.vi"("Application ref in"=w479, "Get data (F)"=TRUE, "Error in (no error)"=w478) -> ("Application ref out"=w477:refnum<vi>, "Data"=w474:sgl[][], "Parameters"=w475:sgl[], "Error out"=w476:errorcluster)  [unwired: 8 in, 1 out]
              }
              frame 1 {
                n188 = call <userlib>:"Z-Spectroscopy Start.vi"("Application ref in"=w482, "Get data (F=False)"=TRUE ("Get Data (F)"), "error in (no error)"=w481) -> ("Application ref out"=w483:refnum<vi>, "Data"=w487:sgl[][], "Parameters"=w486:sgl[], "error out"=w484:errorcluster)  [unwired: 8 in, 1 out]
              }
            }
            n189 = Delete From Array(array=w470, length=1, index (row)=0 ("index")) -> (array with subset deleted=w468:sgl[][])  [unwired: 1 in, 1 out]
            n190 = Write to Binary File(file (use dialog)=w473, data=w469, error in=w463, 5:FALSE ("prepend array or string size? (T)")) -> (refnum out=w472:refnum<file>, error out=w462:errorcluster)  [unwired: 2 in, 1 out]
            n191 = Write to Binary File(file (use dialog)=w472, data=w468, error in=w462, 5:FALSE ("prepend array or string size? (T)")) -> (refnum out=w471:refnum<file>, error out=w454:errorcluster)  [unwired: 2 in, 1 out]
            n192 = Increment(x=w461) -> (x+1=w460:i32)
            n193 = Merge Errors(w455, w454) -> (w453:errorcluster)
          }
        }
        n194 = Get Date/Time In Seconds() -> (seconds since 1Jan1904=w246:timestamp)
        n195 = local read "total Points"() -> (w252:i32)
        n196 = Subtract(x=w246, y=w251) -> (x-y=w250:dbl)
        n197 = Divide(x=w249, y=w252) -> (x/y=w255:dbl)
        n198 = Divide(x=w250, y=w249) -> (x/y=w248:dbl)
        n199 = Subtract(x=w252, y=w249) -> (x-y=w247:i32)
        n200 = Multiply(x=w248, y=w247) -> (x*y=w245:dbl)
        "remaining" <- w245
        n201 = Multiply(x=w255, y=100.0) -> (x*y=→"Progress":dbl)
        n202 = Add(x=w246, y=w245) -> (x+y=→"ETA":timestamp)
      }
      frame "end" {
        n203 = Close File(refnum=w544) -> ()  [unwired: 1 in, 2 out]
        n204 = local write "Status"("finishing" ("Status")) -> ()
        n205 = Bundle(w549, w549) -> (w571:cluster{sgl[][], sgl[][]})  [unwired: 1 in]
        n206 = Close File(refnum=w542) -> (path=w541:path)  [unwired: 1 in, 1 out]
        n207 = call "STSGrid.vi"("Binary Spectroscopy File"=w541) -> ()  [unwired: 11 in]
        n208 = Build Array(w571) -> (w570:cluster{sgl[][], sgl[][]}[])
        n209 = Unbundle By Name(w559) -> ("center X (m)"=w557:sgl, "center Y (m)"=w556:sgl, "angle (deg)"=w555:sgl, "width (m)"=w554:sgl, "height (m)"=w553:sgl)
        n210 = Bundle By Name(cluster=T6 {"center X"=0.0, "center Y"=0.0, "angle"=0.0, "width"=0.0, "height"=0.0, "# pixels"=0, "# lines"=0} ("Scanfield"), "center X"=w557, "center Y"=w556, "angle"=w555, "width"=w554, "height"=w553, "# lines"=w550, "# pixels"=w551) -> (w552:T6)
        n211 = Get Date/Time In Seconds() -> (seconds since 1Jan1904=w526:timestamp)
        n212 = Strip Path(path=w530) -> (stripped path=w563:path, name=w562:string)
        n213 = Bundle By Name(cluster=T8 {"up/down"=FALSE, "time/line"=0.0, "start time"=timestamp(0 s since 1904-01-01), "end time"=timestamp(0 s since 1904-01-01)} ("Scan param"), "up/down"=TRUE, "time/line"=sgl nan ("input 7"), "start time"=w567, "end time"=w526) -> (w566:T8)
        n214 = Bundle("stripped path"=w563, "name"=w562) -> (w561:cluster{"stripped path":path, "name":string})  [unwired: 1 in]
        n215 = call <userlib>:"Save sxm File.vi"("Auto file naming? (T)"=FALSE, "Scanfield"=w552, "Scan param"=w566, "error in (no error)"=w560, "Channels data"=w570, "Channels config"=T7 [{"Name"="Z (m)", "Calibration"=1.0, "Offset"=0.0, "Channel index"=0}], "Filename control"=w561) -> ("error out"=w536:errorcluster)  [unwired: 2 in, 2 out]
        n216 = Strip Path(path=w530) -> (stripped path=w540:path)  [unwired: 1 out]
        n217 = call <userlib>:"Get Session Path.vi"("error in (no error)"=w536, "Application ref in"=w535) -> ("error out"=w532:errorcluster, "Session path"=w534:path, "Application ref out"=w519:refnum<vi>)  [unwired: 7 in]
        n218 = Strip Path(path=w540) -> (stripped path=w539:path)  [unwired: 1 out]
        n219 = Path To String(path=w539) -> (string=w537:string)
        n220 = call "SXM.vi"("Path"=w534, "Delete"=FALSE, "error in"=w532) -> ("error out"=w531:errorcluster)  [unwired: 7 in]
        n221 = call <userlib>:"BiasSpectroscopy SetProperties.vi"("Application ref in"=w519, "Z-Controller hold (no change)"=enum16{"no change", "on", "off"}."on") -> ("Application ref out"=w517:refnum<vi>)  [unwired: 12 in, 1 out]
        n222 = Format Date/Time String(time format string (%c)=" Finished at %y%m%d - %H%M%S ", seconds (now)=w526) -> (date/time string=w525:string)  [unwired: 1 in]
        n223 = call "ChangeSessionV2.vi"("error in (no error)"=w531, "Session"=w537) -> ("error out"=w509:errorcluster)
        n224 = Path To String(path=w530) -> (string=w529:string)
        n225 = call <userlib>:"TipLift Set.vi"("TipLift (m)"=sgl 0.0, "Application ref in"=w517) -> ("Application ref out"=w514:refnum<vi>)  [unwired: 8 in, 1 out]
        n226 = Search and Replace String(input string="Email when finished", search string="@") -> (number of replacements=w521:i32)  [unwired: 6 in, 3 out]
        n227 = local read "Imaging Current"() -> (w494:dbl)
        n228 = local read "Imaging Bias"() -> (w510:dbl)
        n229 = local read "zFile"() -> (w508:refnum<file>)
        n230 = call "move2mark (SubVI).vi"("Application in"=w514) -> ("Application out"=w496:refnum<vi>)  [unwired: 10 in]
        n231 = call <userlib>:"Z-Ctrl Setpoint Set.vi"("Z Controller setpoint"=w494, "Application ref in"=w496) -> ("Application ref out"=w495:refnum<vi>)  [unwired: 8 in, 1 out]
        n232 = Concatenate Strings(w529, "\r\n", w525) -> (w528:string)
        n233 = Greater Than 0?(x=w521) -> (x > 0?=w520:bool)
        n234 = Close File(refnum=w508, error in=w509) -> (error out=w504:errorcluster)  [unwired: 1 out]
        n235 = case shown="True" w520 {
          tunnel: w504 -> [w576 w581]
          tunnel: w528 -> [_ w579]
          tunnel: "Email when finished" -> [_ w578]
          tunnel: [w576 w577] -> w500
          frame False {
          }
          frame True {
            n236 = call "Send Email"("error in"=w581, "Message"=w579, "Subject"="Grid Finished", "Recipients"=w578) -> ("error out"=w577:errorcluster)  [unwired: 7 in]
          }
        }
        n237 = call <userlib>:"Voltage Set.vi"("Error in (no error)"=w500, "Bias (V)"=w510, "Application ref in"=w495) -> ("Error out"=w503:errorcluster, "Application ref out"=w511:refnum<vi>)  [unwired: 7 in]
        n238 = call <userlib>:"Ctrl-on_off Set.vi"("error in (no error)"=w503, "Z Controller ON/OFF"=TRUE, "Application ref in"=w511) -> ("error out"=w502:errorcluster, "Application ref out"=w513:refnum<vi>)  [unwired: 7 in]
        n239 = call <userlib>:"Point Erase.vi"("Application ref in"=w513, "Point index (-1=All points)"=0, "error in (no error)"=w502) -> ("Application ref out"=w506:refnum<vi>, "error out"=w501:errorcluster)  [unwired: 11 in]
        n240 = call "PLL_On_Off (SubVI).vi"("error in (no error)"=w501, "Output ON/OFF (F=OFF)"=FALSE, "Application in"=w506) -> ("error out"=w499:errorcluster, "Application out"=w507:refnum<vi>)  [unwired: 7 in]
        n241 = case shown="False" "MultiGrid" {
          tunnel: w499 -> [w573 w575]
          tunnel: [w573 w574] -> w498
          frame False {
          }
          frame True {
            n242 = call "CallMultiGrid.vi"("error in (no error)"=w575) -> ("error out"=w574:errorcluster)  [unwired: 10 in]
          }
        }
      }
    }
    "Error out" <- w36
    "Points taken" <- w10
    "X Offset" <- w9
    "Y Offset" <- w8
  }
